vi "GetCurrentProtocol.vi"() -> (2 "protocol name":string)   [LabVIEW 2018]
uses:
  <vilib>/addons/_JKI.lib/REST Client/classes/REST Client/REST Client.lvclass
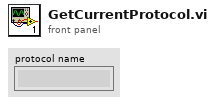
[diagram p1: front panel]
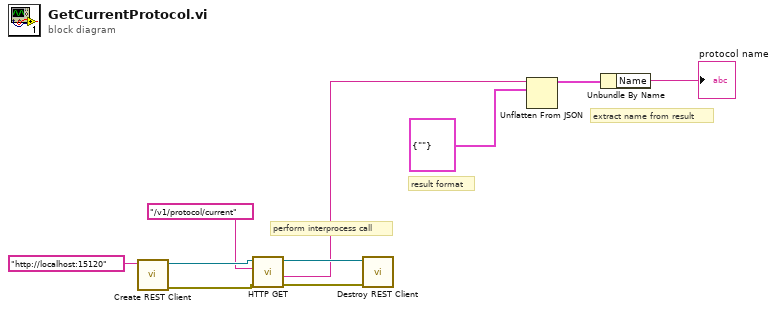
[diagram p0: block diagram]
diagram:
  # "extract name from result"
  # "result format"
  # "perform interprocess call"
  n1 = call <vilib>:"Create REST Client.vi"("Base URL"="http://localhost:15120") -> ("error out"=w8:errorcluster, "REST Client out"=w10:refnum<class "REST Client.lvclass">)  [unwired: 9 in]
  n2 = call-dynamic "HTTP GET.vi"("error in (no error)"=w8, "Path"="/v1/protocol/current", "REST Client in"=w10) -> ("error out"=w7:errorcluster, "Response body"=w2:string, "REST Client out"=w9:refnum<class "REST Client.lvclass">)  [unwired: 3 in, 3 out]
  n3 = call-dynamic "Destroy REST Client.vi"("error in (no error)"=w7, "REST Client in"=w9) -> ()  [unwired: 9 in, 1 out]
  n4 = Unflatten From JSON(JSON string=w2, type and defaults=cluster{"Name":string} {"Name"=""}) -> (value=w1:cluster{"Name":string})  [unwired: 5 in, 1 out]
  n5 = Unbundle By Name(w1) -> ("Name"=→"protocol name":string)
